vi "SynchIO.MyTest.vi"() -> ()   [LabVIEW 2016, in "SynchIO.lvclass"]
doc: "JKI State Machine Objects (SMO) 1.0.0.5\nJKI - JKI\nCopyright (c) 2016, JKI"
uses:
  SynchIO.lvclass
  <vilib>/JKI/JKI SMO/SMO/SMO.lvclass
  <vilib>/JKI/JKI SMO/SMO/Typedefs/SMOState --Enum.ctl
  SynchIO.USB4431/SynchIO.USB4431.lvclass
  C:/Program Files (x86)/National Instruments/LabVIEW 2016/vi.lib/JKI/JKI SMO/SMO/SMO.lvclass
  I:/levy_SVN/lockin/branches/jlevy/SMO/SynchIO/SynchIO.lvclass
panel:
  in  "AI task":tag[](array[tag])
  in  "AO Task":tag[](array[tag])
  in  "AI/AO Config":T1={"AI Configuration"=[], "AO Configuration"=[], "sampling info"={"Fs"=0.0, "#s"=0.0}, "AO"={"AO amp (V)"=[0.1, 0.09, 0.08, 0.07, 0.06, 0.05, 0.04, 0.03], "AO DC (V)"=[0.0, 0.0, 0.0, 0.0, 0.0, 0.0, 0.0, 0.0], "AO f (Hz)"=[13.0, 13.0, 13.0, 13.0, 13.0, 13.0, 13.0, 13.0], "AO phi (deg)"=[0.0, 0.0, 0.0, 0.0, 0.0, 0.0, 0.0, 0.0], "function"=[enum."Sine Wave", enum."Sine Wave", enum."Sine Wave", enum."Sine Wave", enum."Sine Wave", enum."Sine Wave", enum."Sine Wave", enum."Sine Wave"]}} {"AO"."AO DC (V)" format="%#_6p"; "AO"."AO amp (V)" format="%#_6p"}
  in  "AO Array":waveform(dbl)[](array[waveform])=[{"t0"=timestamp(3565884128.737216 s since 1904-01-01), "dt"=9.766769543305856e-06, "Y"=array[7876 elements]}]
  out "Input Signals":waveform(dbl)[](array[waveform])
  in  "4431?":bool=TRUE
  in  "IO Info":T2={"AI task"=[], "sampling info"={"Fs"=1000.0, "#s"=1000.0}, "AO Array"=[], "AO Task"=[], "Reset"=FALSE} {"sampling info"."Fs" format="%.2p"}
  out "Old Value":string
  out "New Value":string
  in  "Send":bool
  in  "Data":string
  out "error out":errorcluster
  in  "Stop":bool
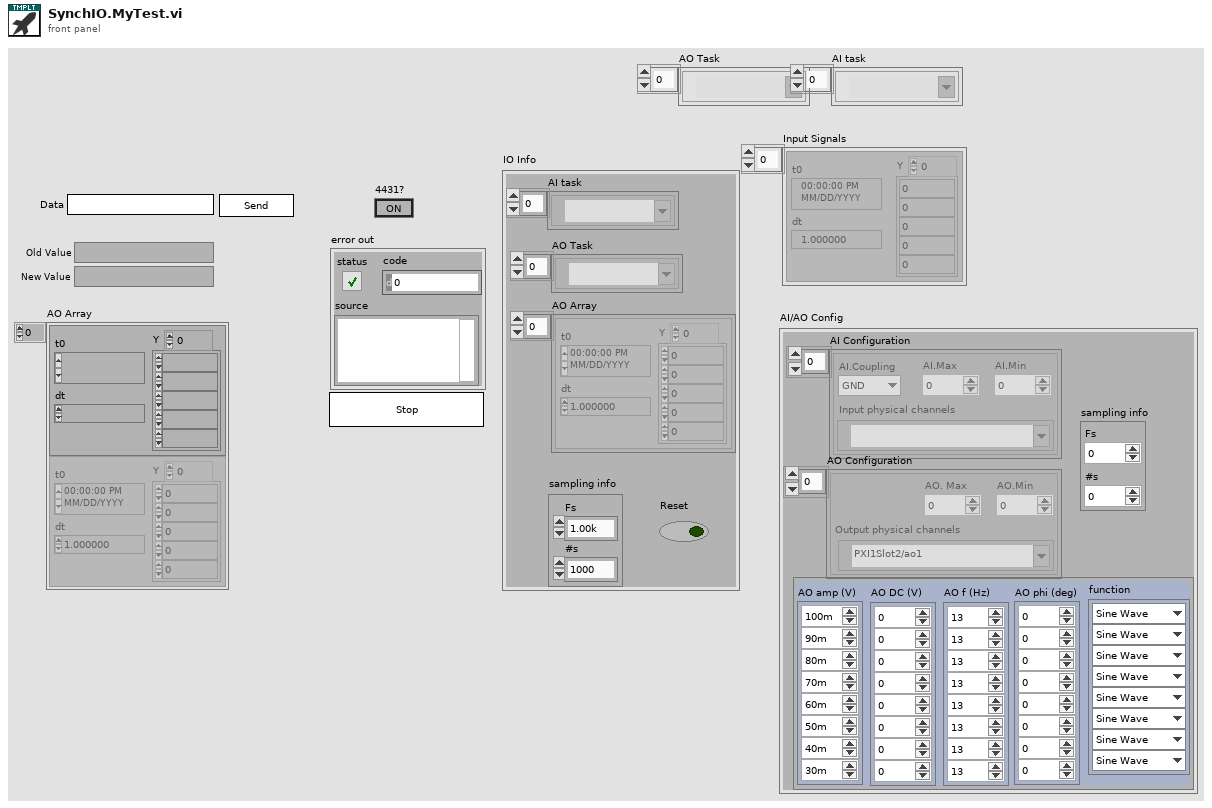
[diagram p1: front panel]
types:
  T1 = cluster{"AI Configuration":cluster{"AI.Coupling":enum16{"AC", "DC", "GND"}, "AI.Max":dbl, "AI.Min":dbl, "Input physical channels":tag}[], "AO Configuration":cluster{"Output physical channels":tag, "AO. Max":dbl, "AO.Min":dbl}[], "sampling info":cluster{"Fs":dbl, "#s":dbl}, "AO":cluster{"AO amp (V)":dbl[], "AO DC (V)":dbl[], "AO f (Hz)":dbl[], "AO phi (deg)":dbl[], "function":enum16{"Sine Wave", "Triangle Wave", "Square Wave", "Sawtooth Wave"}[]}}
  T2 = cluster{"AI task":tag[], "sampling info":cluster{"Fs":dbl, "#s":dbl}, "AO Array":waveform(dbl)[], "AO Task":tag[], "Reset":bool}
  T3 = typedef "SynchIO.lvclass/PublicEvents--Cluster.ctl" = cluster{"Data Changed":refnum<user-event>}
  T4 = cluster{"AI.Coupling":enum16{"AC", "DC", "GND"}, "AI.Max":dbl, "AI.Min":dbl, "Input physical channels":tag}[]
  T5 = cluster{"Output physical channels":tag, "AO. Max":dbl, "AO.Min":dbl}[]
  T6 = typedef "SMO.lvclass/Public Events.ctl" = cluster{"Error":refnum<user-event>, "State":refnum<user-event>}
  T7 = typedef "SMO.lvclass/SMOState --Enum.ctl" = enum16{"unknown", "Created", "Started", "Stopped"}
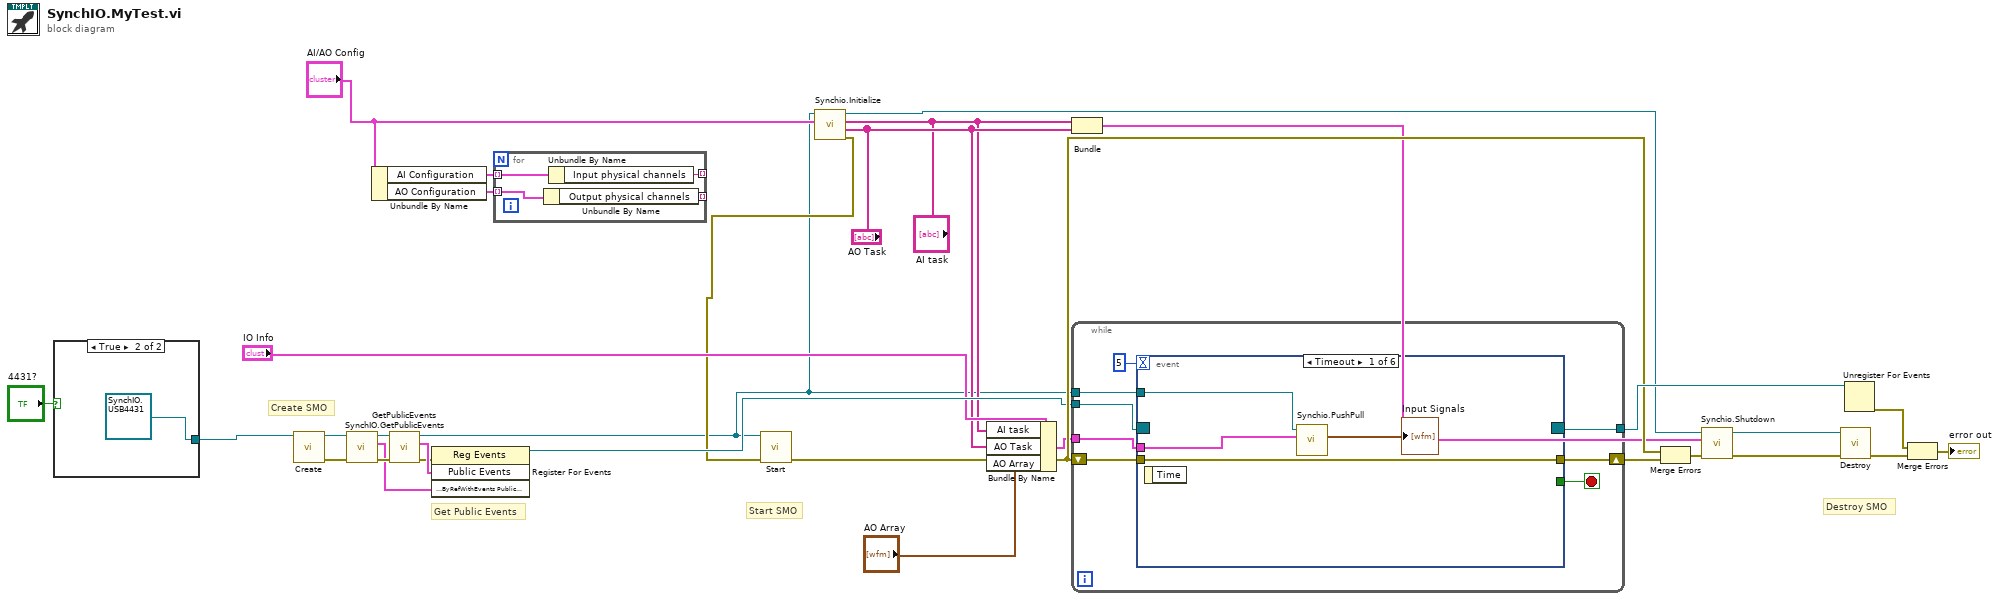
[diagram p0: block diagram]
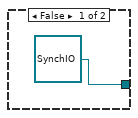
[diagram p2: hidden frame]
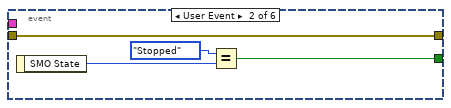
[diagram p3: hidden frame]
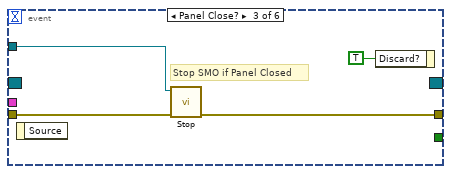
[diagram p4: hidden frame]
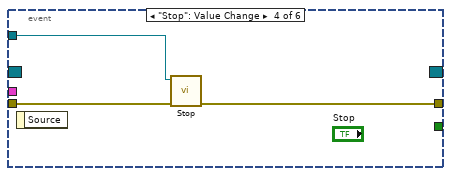
[diagram p5: hidden frame]
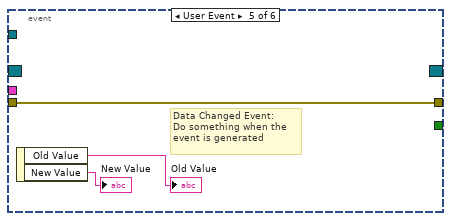
[diagram p6: hidden frame]
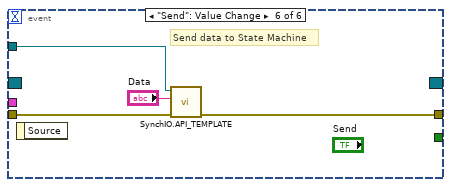
[diagram p7: hidden frame]
diagram:
  # "Get Public Events"
  # "Start SMO"
  # "Destroy SMO"
  # "Create SMO"
  n1 = case shown="True" "4431?" {
    tunnel: [refnum<class "SynchIO.lvclass"> refnum ("SMO.Template.lvclass") refnum<class "SynchIO.USB4431.lvclass"> refnum ("SynchIO.USB4431.lvclass")] -> w8
    frame False {
    }
    frame True {
    }
  }
  n2 = call <vilib>:"Create.vi"("SMO"=w8) -> ("error out"=w22:errorcluster, "SMO out"=w20:refnum<class "SynchIO.lvclass">)  [unwired: 8 in, 1 out]
  n3 = call "SynchIO.GetPublicEvents.vi"("error in (no error)"=w22, "SynchIO"=w20) -> ("error out"=w21:errorcluster, "SMO.ByRefWithEvents Public Events"=w18:T3, "SynchIO out"=w19:refnum<class "SynchIO.lvclass">)  [unwired: 7 in]
  n4 = Unbundle By Name("AI/AO Config") -> ("AI Configuration"=w4:T4, "AO Configuration"=w3:T5)
  n5 = call <vilib>:"GetPublicEvents.vi"("error in (no error)"=w21, "SMO"=w19) -> ("error out"=w24:errorcluster, "Public Events"=w25:T6, "SMO out"=w1:refnum<class "SynchIO.lvclass">)  [unwired: 7 in]
  n6 = register-events(error in=w24, w25, w18) -> (reference out=w23:refnum<event-registration>)  [unwired: 1 in, 1 out]
  n7 = for {
    tunnel: w4 -> [w37] mode=indexing
    tunnel: w3 -> [w36] mode=indexing
    tunnel: [w35] -> _ mode=indexing
    tunnel: [w34] -> _ mode=indexing
    n8 = Unbundle By Name(w36) -> ("Output physical channels"=w34:tag)
    n9 = Unbundle By Name(w37) -> ("Input physical channels"=w35:tag)
  }
  n10 = call-dynamic "Synchio.Initialize.vi"("AO Task"="AO Task", "AI task"="AI task", "AI/AO Config"="AI/AO Config", "SynchIO in"=w1) -> ("error out"=w2:errorcluster, "SynchIO out"=w14:refnum<class "SynchIO.lvclass">)  [unwired: 6 in]
  n11 = call <vilib>:"Start.vi"("error in (no error)"=w2, "SMO"=w1) -> ("error out"=w26:errorcluster)  [unwired: 8 in, 1 out]
  n12 = Bundle By Name(cluster="IO Info", "AI task"="AI task", "AO Task"="AO Task", "AO Array"="AO Array") -> (w16:T2)
  n13 = Bundle("AI task"="AI task", "AO Task"="AO Task") -> (w11:cluster{"AI task":tag[], "AO Task":tag[]})  [unwired: 1 in]
  n14 = while {
    shift-right: [w44] -> w30
    shift-left: w26 -> [w43]
    tunnel: w23 -> [w42]
    tunnel: [w41] -> w31
    tunnel: w1 -> [w40]
    tunnel: w16 -> [w38]
    stop <- w45 stop-if-true
    n15 = event shown="[0] Timeout" {
      selector: w42 -> [_ _ _ _ _ _]
      dyn-events: [_ _ _ _ _ _] -> w41
      timeout: 5 -> [_ _ _ _ _ _]
      tunnel: [_ w50 _ _ _ _] -> w45
      tunnel: w40 -> [w48 _ w57 w60 _ w67]
      tunnel: [w49 w53 w56 w59 w63 w64] -> w44
      tunnel: w43 -> [w49 w53 w55 w58 w63 w65]
      tunnel: w38 -> [w47 _ _ _ _ _]
      event Timeout {
        n16 = event-data() -> ()  [unwired: 1 in, 1 out]
        n17 = call-dynamic "Synchio.PushPull.vi"("IO Info"=w47, "SynchIO in"=w48) -> ("Input Signals"=→"Input Signals":waveform(dbl)[])  [unwired: 7 in, 2 out]
      }
      event User Event {
        n18 = event-data() -> ("SMO State"=w52:T7)  [unwired: 1 in]
        n19 = Equal?(x=SMOState_--Enum."Stopped", y=w52) -> (x = y?=w50:bool)
      }
      event Panel Close? {
        # "Stop SMO if Panel Closed"
        n20 = event-data() -> ()  [unwired: 1 in, 1 out]
        n21 = call <vilib>:"Stop.vi"("error in (no error)"=w55, "SMO"=w57) -> ("error out"=w56:errorcluster)  [unwired: 8 in, 1 out]
        n22 = event-data("Discard?"=TRUE ("OK")) -> ()  [unwired: 1 in, 1 out]
      }
      event "Stop": Value Change {
        n23 = event-data() -> ()  [unwired: 1 in, 1 out]
        n24 = call <vilib>:"Stop.vi"("error in (no error)"=w58, "SMO"=w60) -> ("error out"=w59:errorcluster)  [unwired: 8 in, 1 out]
      }
      event User Event {
        # "Data Changed Event:\nDo something when the\nevent is generated"
        n25 = event-data() -> ("Old Value"=→"Old Value":string, "New Value"=→"New Value":string)  [unwired: 1 in]
      }
      event "Send": Value Change {
        # "Send data to State Machine"
        n26 = event-data() -> ()  [unwired: 1 in, 1 out]
        n27 = call "SynchIO.API_TEMPLATE.vi"("error in (no error)"=w65, "myData"="Data", "SynchIO"=w67) -> ("error out"=w64:errorcluster)  [unwired: 6 in, 2 out]
      }
    }
  }
  n28 = Merge Errors(w26, w30) -> (w13:errorcluster)
  n29 = call-dynamic "Synchio.Shutdown.vi"("error in (no error)"=w13, "AIAO Tasks"=w11, "SynchIO in"=w14) -> ("error out"=w12:errorcluster, "SynchIO out"=w15:refnum<class "SynchIO.lvclass">)  [unwired: 7 in]
  n30 = call <vilib>:"Destroy.vi"("error in (no error)"=w12, "SMO"=w15) -> ("error out"=w27:errorcluster)  [unwired: 9 in]
  n31 = Unregister For Events(event registration refnum=w31) -> (error out=w29:errorcluster)  [unwired: 1 in]
  n32 = Merge Errors(w29, w27) -> (→"error out":errorcluster)
